vi "FastWriter_V01_Working.vi"() -> ()   [LabVIEW 2012]
uses:
  WVD-MCSupdate/WVDNewArchitectureUpdate/WVD_Architecture_Update/TypeDefinitions.llb/TypeDef_MPDUnitID.ctl
panel:
  out "Receive Buffer Size":u32
  out "WriteCount":i32
  out "LoopCount":i32
  out "error out":errorcluster
  in  "stop":bool
  in  "MPDUnitID":T1=enum."MPD#01"
  in  "DataBasePath":string="C:\\Users\\h2odial\\WVD-MCSupdate\\WVDNewArchitectureUpdate\\WVD_Architecture_Update\\Data\\TCSPC\\"
  in  "FileBaseNameIn":string="TCSPCFastData"
  in  "UDP Port":u16=54002
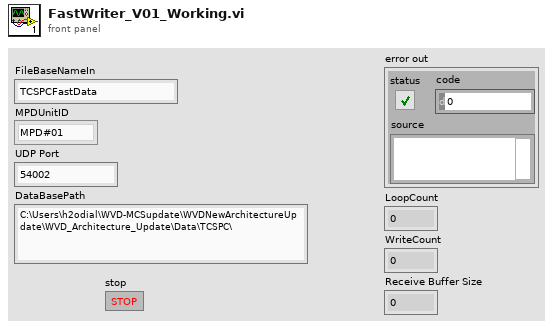
[diagram p1: front panel]
types:
  T1 = typedef "TypeDef_MPDUnitID.ctl" = enum8{"Unknown", "MPD#01", "MPD#02", "MPD#03", "MPD#04", "MPD#05"}
  T2 = enum16{"open", "replace", "create", "open or create", "replace or create", "replace or create with confirmation"}
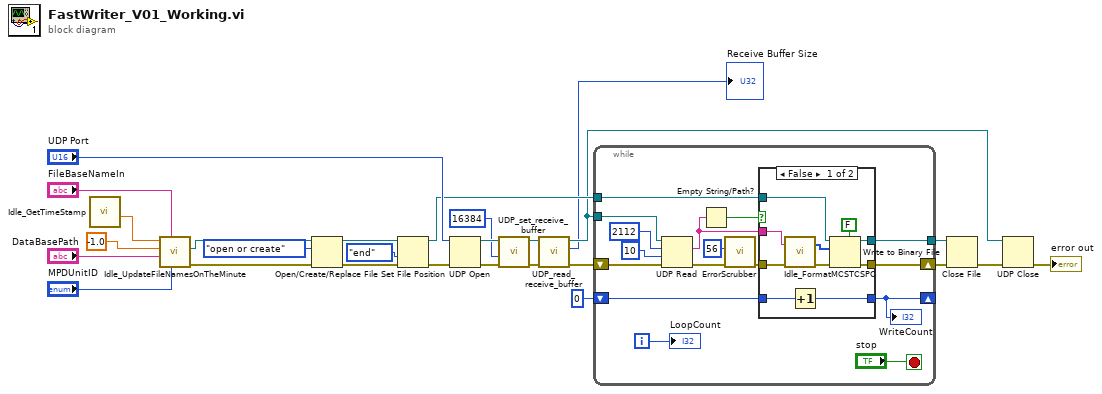
[diagram p0: block diagram]
diagram:
  n1 = call "Idle_GetTimeStamp.vi"() -> ("Fractional Hours"=w25:dbl)  [unwired: 11 in]
  n2 = call "Idle_UpdateFileNamesOnTheMinute.vi"("MPDUnitID"="MPDUnitID", "FileBaseNameIn"="FileBaseNameIn", "DataBasePathIn"="DataBasePath", "FileUpdateTimeIn"=-1.0, "CurrentTime"=w25) -> ("ErrorOur"=w17:errorcluster, "WritePathOut"=w16:path)  [unwired: 3 in, 2 out]
  n3 = Open/Create/Replace File(file path (use dialog)=w16, error in=w17, operation (0:open)=T2."open or create") -> (refnum out=w19:refnum<file>, error out=w18:errorcluster)  [unwired: 3 in, 1 out]
  n4 = Set File Position(refnum=w19, from (0:start)=enum16{"start", "end", "current"}."end", error in=w18) -> (refnum out=w14:refnum<file>, error out=w15:errorcluster)  [unwired: 1 in]
  n5 = UDP Open(8:w15, 11:"UDP Port") -> (port=w7:refnum<k16>, 0:w8:errorcluster)  [unwired: 3 in, 1 out]
  n6 = call "UDP_set_receive_buffer.vi"("error in (no error)"=w8, "Receive Buffer Size"=u32 16384, "connection ID"=w7) -> ("error out"=w5:errorcluster, "connection ID out"=w3:refnum<k16>)  [unwired: 6 in]
  n7 = call "UDP_read_receive_buffer.vi"("error in (no error)"=w5, "connection ID"=w3) -> ("error out"=w4:errorcluster, "Receive Buffer Size"=→"Receive Buffer Size":u32, "connection ID out"=w2:refnum<k16>)  [unwired: 5 in]
  n8 = while {
    tunnel: w14 -> [w36]
    shift-right: [w33] -> _
    shift-left: 0 -> [w34]
    shift-right: [w31] -> w12
    shift-left: w4 -> [w32]
    tunnel: [w30] -> w11
    tunnel: w2 -> [w29]
    i -> [w28]
    stop <- "stop" stop-if-true
    n9 = UDP Read(connection ID=w29, max size (548)=2112, timeout ms (25000)=10, 8:w32) -> (data out=w40:string, error out=w42:errorcluster)  [unwired: 3 out]
    n10 = Empty String/Path?(string/path=w40) -> (empty?=w39:bool)
    n11 = call "ErrorScrubber.vi"("error in (no error)"=w42, "y"=56) -> ("error out"=w41:errorcluster)  [unwired: 8 in, 1 out]
    n12 = case shown="False" w39 {
      tunnel: w41 -> [w53 w56]
      tunnel: w36 -> [w52 w55]
      tunnel: [w51 w55] -> w30
      tunnel: [w50 w56] -> w31
      tunnel: w40 -> [w49 _]
      tunnel: w34 -> [w48 w54]
      tunnel: [w47 w54] -> w33
      frame False {
        n13 = call "Idle_FormatMCSTCSPC.vi"("ErrorIn"=w53, "UDPResponse"=w49) -> ("ErrorOut"=w45:errorcluster, "ByteArray"=w44:u8[])
        n14 = Increment(x=w48) -> (x+1=w47:i32)
        n15 = Write to Binary File(file (use dialog)=w52, data=w44, error in=w45, 5:FALSE ("prepend array or string size? (T)")) -> (refnum out=w51:refnum<file>, error out=w50:errorcluster)  [unwired: 2 in, 1 out]
      }
      frame True {
      }
    }
    "WriteCount" <- w33
    "LoopCount" <- w28
  }
  n16 = Close File(refnum=w11, error in=w12) -> (error out=w10:errorcluster)  [unwired: 1 out]
  n17 = UDP Close(connection ID=w2, 8:w10) -> (error out=→"error out":errorcluster)  [unwired: 1 out]
